vi "COMPORT-SearchCOMsForDevice.vi"(8 "error in (no error)":errorcluster, 11 "SearchSTR":string="ASRL?*INSTR") -> (0 "error out":errorcluster, 2 "Device COM found?":bool, 3 "COM-out":refnum<visa-resource-name>)   [LabVIEW 2020]
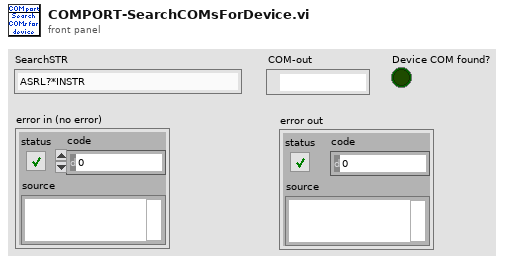
[diagram p1: front panel]
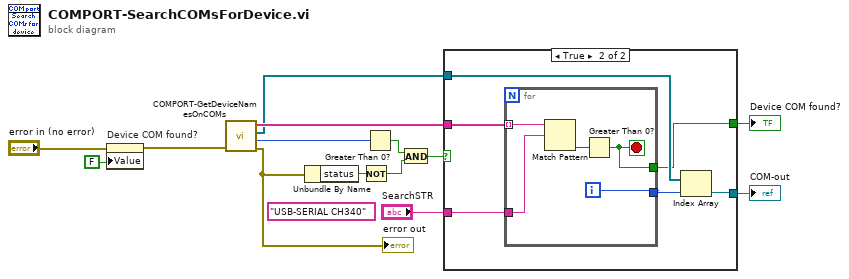
[diagram p0: block diagram]
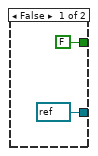
[diagram p2: hidden frame]
diagram:
  (unwired) "USB-SERIAL CH340" ("expression (\"?*\")")
  n1 = property on="Device COM found?" class="Bool (strict)"(error in="error in (no error)", "Value"=FALSE ("Device found?")) -> (error out=w3:errorcluster)  [unwired: 1 in, 1 out]
  n2 = call "COMPORT-GetDeviceNamesOnCOMs.vi"("error in (no error)"=w3) -> ("error out"=w5:errorcluster, "#Resources"=w10:u32, "COMs Arr"=w7:refnum<visa-resource-name>[], "COMDeviceList Arr"=w14:string[])  [unwired: 7 in]
  "error out" <- w5
  n3 = Unbundle By Name(w5) -> ("status"=w11:bool)
  n4 = Not(x=w11) -> (.not. x?=w12:bool)
  n5 = Greater Than 0?(x=w10) -> (x > 0?=w13:bool)
  n6 = And(x=w13, y=w12) -> (x .and. y?=w9:bool)
  n7 = case shown="True" w9 {
    tunnel: w14 -> [_ w21]
    tunnel: "SearchSTR" -> [_ w22]
    tunnel: w7 -> [_ w19]
    tunnel: [refnum<visa-resource-name> refnum ("VISA resource name out") w18] -> w6
    tunnel: [FALSE w17] -> w4
    frame False {
    }
    frame True {
      n8 = for {
        tunnel: w21 -> [w27] mode=indexing
        tunnel: w22 -> [w26]
        tunnel: [w24] -> w20
        tunnel: [w23] -> w17
        i -> [w24]
        stop <- w23 stop-if-true
        n9 = Match Pattern(string=w27, regular expression=w26) -> (offset past match=w25:i32)  [unwired: 1 in, 3 out]
        n10 = Greater Than 0?(x=w25) -> (x > 0?=w23:bool)
      }
      n11 = Index Array(array=w19, index=w20) -> (element=w18:refnum<visa-resource-name>)
    }
  }
  "COM-out" <- w6
  "Device COM found?" <- w4
